vi "Excel___Create Channel Grouping.vi"(0 "Sheets Ref In":refnum<k7>, 5 "Starting Row":i32, 7 "Units String":string, 9 "Action to Perform":u16(ring) items=["", "Start Calibration", "Continue Calibration", "System Initialization", "System Closeout"], 11 "Error In":errorcluster, 12 "Percent Error(F)":bool, 13 "FS(T)/Reading(F)":bool) -> (4 "Sheets Ref Out":refnum<k7>, 15 "Error Out":errorcluster)   [LabVIEW 2019]
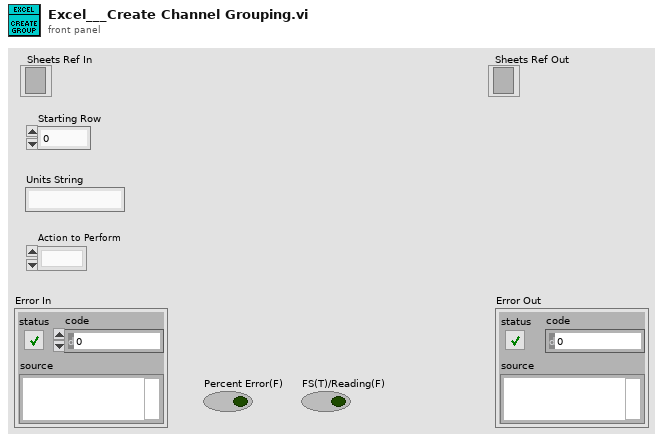
[diagram p1: front panel]
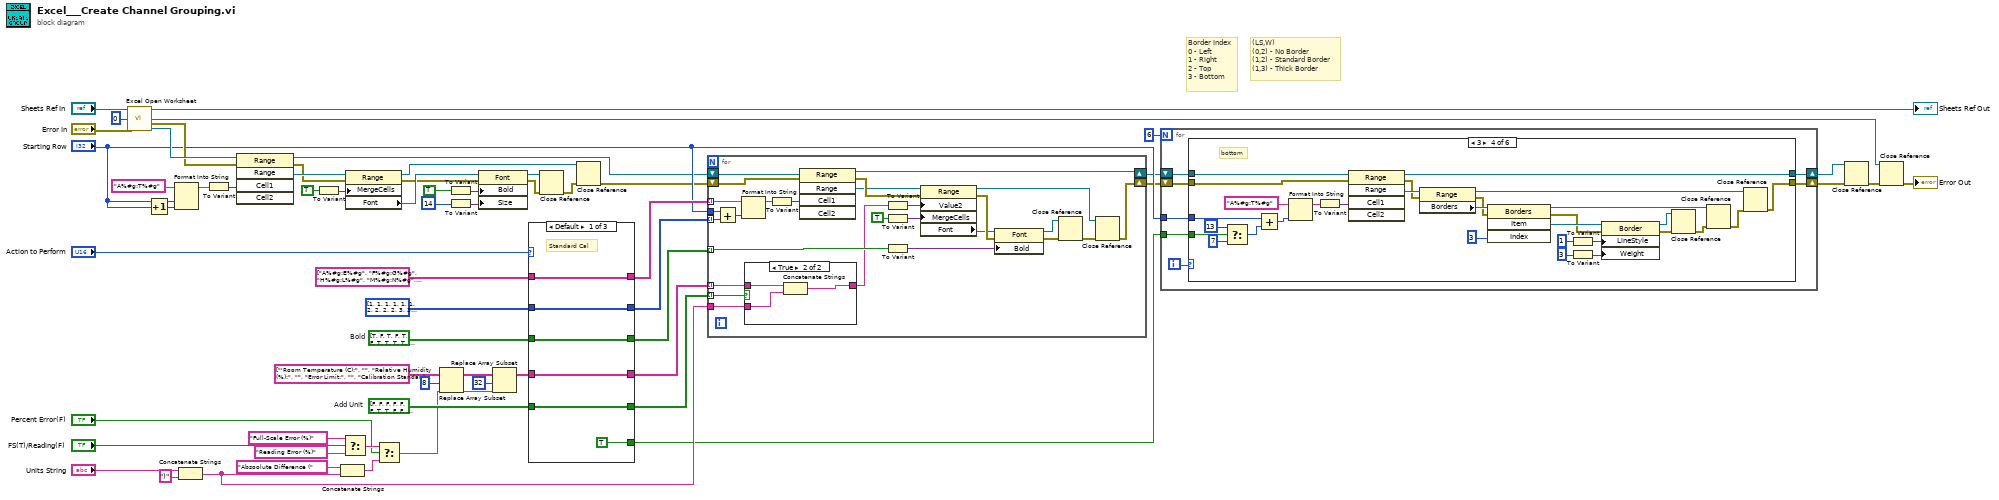
[diagram p0: block diagram]
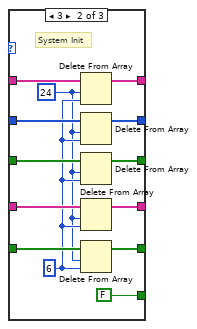
[diagram p3: hidden frame]
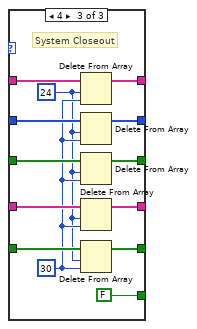
[diagram p4: hidden frame]
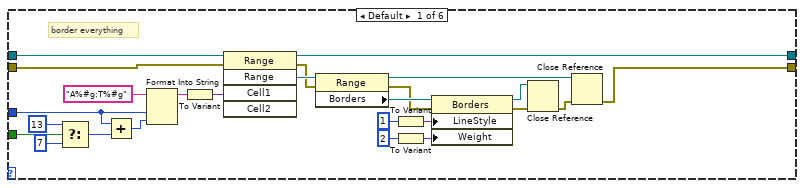
[diagram p5: hidden frame]
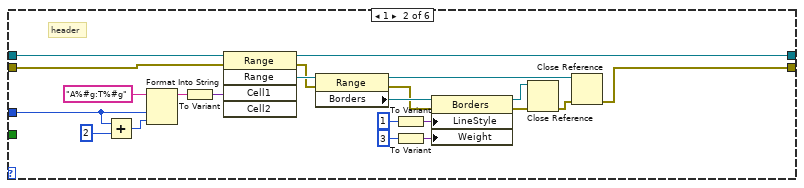
[diagram p6: hidden frame]
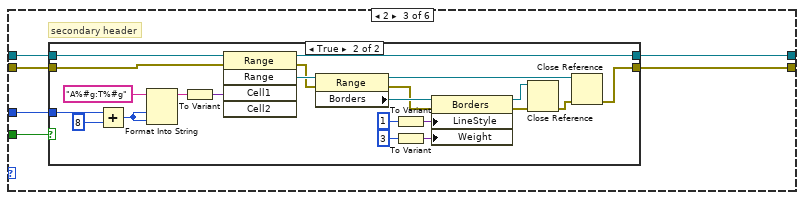
[diagram p7: hidden frame]
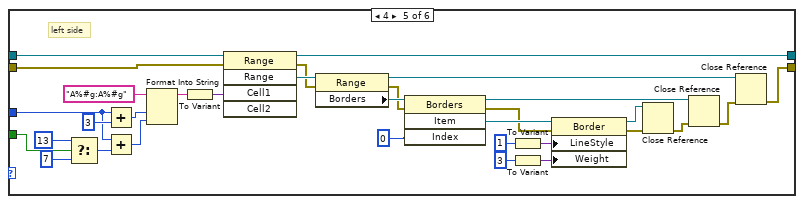
[diagram p9: hidden frame]
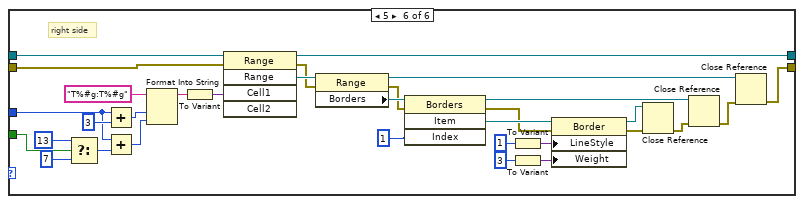
[diagram p10: hidden frame]
diagram:
  w26 = bool[] [FALSE, FALSE, FALSE, FALSE, FALSE, FALSE, TRUE, TRUE, FALSE, FALSE, FALSE, FALSE, FALSE, FALSE, FALSE, FALSE, FALSE, FALSE, FALSE, FALSE, FALSE, FALSE, FALSE, FALSE, FALSE, FALSE, FALSE, FALSE, FALSE, FALSE, TRUE, TRUE, FALSE, FALSE, FALSE, FALSE, FALSE, FALSE, FALSE, FALSE, FALSE, FALSE, FALSE, FALSE, FALSE, FALSE, FALSE, FALSE, FALSE, FALSE, FALSE, FALSE, FALSE, FALSE]  # Add Unit
  w27 = bool[] [TRUE, FALSE, TRUE, FALSE, TRUE, FALSE, TRUE, TRUE, TRUE, TRUE, FALSE, FALSE, FALSE, FALSE, FALSE, FALSE, FALSE, FALSE, FALSE, FALSE, FALSE, FALSE, FALSE, FALSE, FALSE, FALSE, FALSE, FALSE, FALSE, FALSE, TRUE, TRUE, TRUE, TRUE, FALSE, FALSE, FALSE, FALSE, FALSE, FALSE, FALSE, FALSE, FALSE, FALSE, FALSE, FALSE, FALSE, FALSE, FALSE, FALSE, FALSE, FALSE, FALSE, FALSE]  # Bold
  # "(LS,W)\n(0,2) - No Border\n(1,2) - Standard Border\n(1,3) - Thick Border"
  # "Border Index\n0 - Left\n1 - Right\n2 - Top\n3 - Bottom"
  n1 = call "Excel Open Worksheet.vi"("Sheets Ref In"="Sheets Ref In", "Sheet#"=0, "Error In"="Error In") -> ("Sheets Ref Out"=→"Sheets Ref Out":refnum<k7>, "Worksheet Ref Out"=w43:refnum<k7>, "Error Out"=w39:errorcluster, "Cells Ref Out"=w40:refnum<k7>)  [unwired: 9 in]
  n2 = Increment(x="Starting Row") -> (x+1=w61:i32)
  n3 = Format Into String(initial string="A%#g:T%#g", "Starting Row", w61) -> (resulting string=w60:string)  [unwired: 2 in, 1 out]
  n4 = Concatenate Strings("Units String", ")" ("string")) -> (w2:string)
  n5 = To Variant(anything=w60) -> (Variant=w59:variant)
  n6 = invoke class="Range" method="Range"(reference=w40, error in=w39, "Cell1"=w59) -> (reference out=w7:refnum<k7>, error out=w49:errorcluster, "Range"=w58:refnum<k7>)  [unwired: 2 in, 2 out]
  n7 = To Variant(anything=TRUE) -> (Variant=w56:variant)
  n8 = Concatenate Strings("Absoolute Difference (", w2) -> (w15:string)
  n9 = Select(t="Full-Scale Error (%)", s="FS(T)/Reading(F)", f="Reading Error (%)") -> (s? t:f=w16:string)
  n10 = property class="Range"(reference=w58, error in=w49, "MergeCells"=w56) -> (reference out=w34:refnum<k7>, error out=w54:errorcluster, "Font"=w55:refnum<k7>)
  n11 = Select(t=w16, s="Percent Error(F)", f=w15) -> (s? t:f=w14:string)
  n12 = Replace Array Subset(array=string[] ["'Room Temperature (C):", "", "Relative Humidity (%):", "", "Error Limit:", "", "Calibration Standard (", "Reading As Found (", "***placeholder***", "Results", "", "", "", "", "5", "", "", "", "", "10", "", "", "", "", "15", "", "", "", "", "20", "Calibration Standard (", "Reading As Left (", "***placeholder***", "Results", "", "", "", "", "5", "", "", "", "", "10", "", "", "", "", "15", "", "", "", "", "20"], new element=w14, index=8) -> (w13:string[])
  n13 = To Variant(anything=TRUE) -> (Variant=w52:variant)
  n14 = To Variant(anything=14) -> (Variant=w51:variant)
  n15 = property class="Font"(reference=w55, error in=w54, "Bold"=w52, "Size"=w51) -> (reference out=w36:refnum<k7>, error out=w35:errorcluster)
  n16 = Replace Array Subset(array=w13, new element=w14, index=32) -> (w11:string[])
  n17 = case shown="Default" "Action to Perform" {
    tunnel: [w68 w72 w85] -> w25
    tunnel: string[] ["A%#g:E%#g", "F%#g:G%#g", "H%#g:L%#g", "M%#g:N%#g", "O%#g:Q%#g", "R%#g:T%#g", "A%#g:F%#g", "G%#g:L%#g", "M%#g:R%#g", "S%#g:T%#g", "A%#g:F%#g", "G%#g:L%#g", "M%#g:R%#g", "S%#g:T%#g", "A%#g:F%#g", "G%#g:L%#g", "M%#g:R%#g", "S%#g:T%#g", "A%#g:F%#g", "G%#g:L%#g", "M%#g:R%#g", "S%#g:T%#g", "A%#g:F%#g", "G%#g:L%#g", "M%#g:R%#g", "S%#g:T%#g", "A%#g:F%#g", "G%#g:L%#g", "M%#g:R%#g", "S%#g:T%#g", "A%#g:F%#g", "G%#g:L%#g", "M%#g:R%#g", "S%#g:T%#g", "A%#g:F%#g", "G%#g:L%#g", "M%#g:R%#g", "S%#g:T%#g", "A%#g:F%#g", "G%#g:L%#g", "M%#g:R%#g", "S%#g:T%#g", "A%#g:F%#g", "G%#g:L%#g", "M%#g:R%#g", "S%#g:T%#g", "A%#g:F%#g", "G%#g:L%#g", "M%#g:R%#g", "S%#g:T%#g", "A%#g:F%#g", "G%#g:L%#g", "M%#g:R%#g", "S%#g:T%#g"] -> [w68 w76 w94]
    tunnel: [w67 w73 w86] -> w24
    tunnel: i32[] [1, 1, 1, 1, 1, 1, 2, 2, 2, 2, 3, 3, 3, 3, 4, 4, 4, 4, 5, 5, 5, 5, 6, 6, 6, 6, 7, 7, 7, 7, 8, 8, 8, 8, 9, 9, 9, 9, 10, 10, 10, 10, 11, 11, 11, 11, 12, 12, 12, 12, 13, 13, 13, 13] -> [w67 w77 w93]
    tunnel: [w66 w74 w87] -> w22
    tunnel: w27 -> [w66 w78 w92]
    tunnel: [w65 w75 w88] -> w18
    tunnel: w11 -> [w65 w79 w91]
    tunnel: [w64 w80 w89] -> w21
    tunnel: w26 -> [w64 w81 w90]
    tunnel: [TRUE FALSE FALSE] -> w1
    frame Default {
      # "Standard Cal"
    }
    frame 3 {
      w70 = 24 ("length")
      w71 = 6 ("index")
      # "System Init"
      n18 = Delete From Array(array=w76, length=w70, index=w71) -> (array with subset deleted=w72:string[])  [unwired: 1 out]
      n19 = Delete From Array(array=w77, length=w70, index=w71) -> (array with subset deleted=w73:i32[])  [unwired: 1 out]
      n20 = Delete From Array(array=w78, length=w70, index=w71) -> (array with subset deleted=w74:bool[])  [unwired: 1 out]
      n21 = Delete From Array(array=w79, length=w70, index=w71) -> (array with subset deleted=w75:string[])  [unwired: 1 out]
      n22 = Delete From Array(array=w81, length=w70, index=w71) -> (array with subset deleted=w80:bool[])  [unwired: 1 out]
    }
    frame 4 {
      w83 = 24 ("length")
      w84 = 30 ("index")
      # "System Closeout"
      n23 = Delete From Array(array=w94, length=w83, index=w84) -> (array with subset deleted=w85:string[])  [unwired: 1 out]
      n24 = Delete From Array(array=w93, length=w83, index=w84) -> (array with subset deleted=w86:i32[])  [unwired: 1 out]
      n25 = Delete From Array(array=w92, length=w83, index=w84) -> (array with subset deleted=w87:bool[])  [unwired: 1 out]
      n26 = Delete From Array(array=w91, length=w83, index=w84) -> (array with subset deleted=w88:string[])  [unwired: 1 out]
      n27 = Delete From Array(array=w90, length=w83, index=w84) -> (array with subset deleted=w89:bool[])  [unwired: 1 out]
    }
  }
  n28 = Close Reference(reference=w36, error in (no error)=w35) -> (error out=w33:errorcluster)
  n29 = Close Reference(reference=w34, error in (no error)=w33) -> (error out=w6:errorcluster)
  n30 = for {
    tunnel: w25 -> [w121] mode=indexing
    tunnel: "Starting Row" -> [w119]
    tunnel: w24 -> [w118] mode=indexing
    shift-right: [w105] -> w5
    shift-left: w7 -> [w104]
    shift-right: [w103] -> w4
    shift-left: w6 -> [w102]
    tunnel: w22 -> [w99] mode=indexing
    tunnel: w21 -> [w98] mode=indexing
    tunnel: w18 -> [w97] mode=indexing
    tunnel: w2 -> [w95]
    n31 = Add(x=w119, y=w118) -> (x+y=w120:i32)
    n32 = Format Into String(initial string=w121, w120) -> (resulting string=w111:string)  [unwired: 2 in, 1 out]
    n33 = case shown="True" w98 {
      tunnel: w97 -> [w122 w125]
      tunnel: [w122 w124] -> w96
      tunnel: w95 -> [_ w123]
      frame False {
      }
      frame True {
        n34 = Concatenate Strings(w125, w123) -> (w124:string)
      }
    }
    n35 = To Variant(anything=w111) -> (Variant=w112:variant)
    n36 = invoke class="Range" method="Range"(reference=w104, error in=w102, "Cell1"=w112) -> (reference out=w105:refnum<k7>, error out=w117:errorcluster, "Range"=w113:refnum<k7>)  [unwired: 2 in, 2 out]
    n37 = To Variant(anything=w96) -> (Variant=w110:variant)
    n38 = To Variant(anything=TRUE) -> (Variant=w101:variant)
    n39 = To Variant(anything=w99) -> (Variant=w100:variant)
    n40 = property class="Range"(reference=w113, error in=w117, "Value2"=w110, "MergeCells"=w101) -> (reference out=w106:refnum<k7>, error out=w116:errorcluster, "Font"=w115:refnum<k7>)
    n41 = property class="Font"(reference=w115, error in=w116, "Bold"=w100) -> (reference out=w108:refnum<k7>, error out=w109:errorcluster)
    n42 = Close Reference(reference=w108, error in (no error)=w109) -> (error out=w107:errorcluster)
    n43 = Close Reference(reference=w106, error in (no error)=w107) -> (error out=w103:errorcluster)
  }
  n44 = for {
    N: 6 -> [_]
    shift-right: [w132] -> w38
    shift-left: w5 -> [w130]
    tunnel: "Starting Row" -> [w131]
    shift-right: [w129] -> w37
    shift-left: w4 -> [w128]
    tunnel: w1 -> [w126]
    i -> [w127]
    n45 = case shown="3" w127 {
      tunnel: [w155 w178 w185 w239 w269 w301] -> w132
      tunnel: w131 -> [w153 w159 w181 w238 w246 w278]
      tunnel: w130 -> [w151 w177 w184 w237 w267 w299]
      tunnel: [w138 w164 w183 w236 w257 w289] -> w129
      tunnel: w128 -> [w137 w163 w182 w235 w256 w288]
      tunnel: w126 -> [w136 _ w180 w213 w240 w273]
      frame Default {
        # "border everything"
        n46 = Select(t=13 ("y"), s=w136, f=7) -> (s? t:f=w134:i32)
        n47 = Add(x=w153, y=w134) -> (x+y=w154:i32)
        n48 = Format Into String(initial string="A%#g:T%#g", w153, w154) -> (resulting string=w157:string)  [unwired: 2 in, 1 out]
        n49 = To Variant(anything=w157) -> (Variant=w156:variant)
        n50 = invoke class="Range" method="Range"(reference=w151, error in=w137, "Cell1"=w156) -> (reference out=w155:refnum<k7>, error out=w139:errorcluster, "Range"=w150:refnum<k7>)  [unwired: 2 in, 2 out]
        n51 = property class="Range"(reference=w150, error in=w139) -> (reference out=w141:refnum<k7>, error out=w140:errorcluster, "Borders"=w149:refnum<k7>)
        n52 = To Variant(anything=1) -> (Variant=w148:variant)
        n53 = To Variant(anything=2) -> (Variant=w147:variant)
        n54 = property class="Borders"(reference=w149, error in=w140, "LineStyle"=w148, "Weight"=w147) -> (reference out=w142:refnum<k7>, error out=w143:errorcluster)
        n55 = Close Reference(reference=w142, error in (no error)=w143) -> (error out=w144:errorcluster)
        n56 = Close Reference(reference=w141, error in (no error)=w144) -> (error out=w138:errorcluster)
      }
      frame 1 {
        # "header"
        n57 = Add(x=w159, y=2) -> (x+y=w162:i32)
        n58 = Format Into String(initial string="A%#g:T%#g", w159, w162) -> (resulting string=w158:string)  [unwired: 2 in, 1 out]
        n59 = To Variant(anything=w158) -> (Variant=w179:variant)
        n60 = invoke class="Range" method="Range"(reference=w177, error in=w163, "Cell1"=w179) -> (reference out=w178:refnum<k7>, error out=w165:errorcluster, "Range"=w176:refnum<k7>)  [unwired: 2 in, 2 out]
        n61 = property class="Range"(reference=w176, error in=w165) -> (reference out=w167:refnum<k7>, error out=w166:errorcluster, "Borders"=w175:refnum<k7>)
        n62 = To Variant(anything=1) -> (Variant=w174:variant)
        n63 = To Variant(anything=3) -> (Variant=w173:variant)
        n64 = property class="Borders"(reference=w175, error in=w166, "LineStyle"=w174, "Weight"=w173) -> (reference out=w168:refnum<k7>, error out=w169:errorcluster)
        n65 = Close Reference(reference=w168, error in (no error)=w169) -> (error out=w170:errorcluster)
        n66 = Close Reference(reference=w167, error in (no error)=w170) -> (error out=w164:errorcluster)
      }
      frame 2 {
        # "secondary header"
        n67 = case shown="True" w180 {
          tunnel: [w187 w208] -> w185
          tunnel: w184 -> [w187 w207]
          tunnel: [w186 w194] -> w183
          tunnel: w182 -> [w186 w193]
          tunnel: w181 -> [_ w190]
          frame False {
          }
          frame True {
            n68 = Add(x=w190, y=8) -> (x+y=w188:i32)
            n69 = Format Into String(initial string="A%#g:T%#g", w188, w188) -> (resulting string=w189:string)  [unwired: 2 in, 1 out]
            n70 = To Variant(anything=w189) -> (Variant=w209:variant)
            n71 = invoke class="Range" method="Range"(reference=w207, error in=w193, "Cell1"=w209) -> (reference out=w208:refnum<k7>, error out=w195:errorcluster, "Range"=w206:refnum<k7>)  [unwired: 2 in, 2 out]
            n72 = property class="Range"(reference=w206, error in=w195) -> (reference out=w197:refnum<k7>, error out=w196:errorcluster, "Borders"=w205:refnum<k7>)
            n73 = To Variant(anything=1) -> (Variant=w204:variant)
            n74 = To Variant(anything=3) -> (Variant=w203:variant)
            n75 = property class="Borders"(reference=w205, error in=w196, "LineStyle"=w204, "Weight"=w203) -> (reference out=w198:refnum<k7>, error out=w199:errorcluster)
            n76 = Close Reference(reference=w198, error in (no error)=w199) -> (error out=w200:errorcluster)
            n77 = Close Reference(reference=w197, error in (no error)=w200) -> (error out=w194:errorcluster)
          }
        }
      }
      frame 3 {
        # "bottom"
        n78 = Select(t=13 ("y"), s=w213, f=7 ("y")) -> (s? t:f=w210:i32)
        n79 = Add(x=w238, y=w210) -> (x+y=w215:i32)
        n80 = Format Into String(initial string="A%#g:T%#g", w215) -> (resulting string=w234:string)  [unwired: 2 in, 1 out]
        n81 = To Variant(anything=w234) -> (Variant=w233:variant)
        n82 = invoke class="Range" method="Range"(reference=w237, error in=w235, "Cell1"=w233) -> (reference out=w239:refnum<k7>, error out=w223:errorcluster, "Range"=w231:refnum<k7>)  [unwired: 2 in, 2 out]
        n83 = property class="Range"(reference=w231, error in=w223) -> (reference out=w224:refnum<k7>, error out=w220:errorcluster, "Borders"=w222:refnum<k7>)
        n84 = invoke class="Borders" method="Item"(reference=w222, error in=w220, "Index"=3) -> (reference out=w217:refnum<k7>, error out=w214:errorcluster, "Item"=w221:refnum<k7>)  [unwired: 1 in, 1 out]
        n85 = To Variant(anything=1) -> (Variant=w230:variant)
        n86 = To Variant(anything=3) -> (Variant=w229:variant)
        n87 = property class="Border"(reference=w221, error in=w214, "LineStyle"=w230, "Weight"=w229) -> (reference out=w225:refnum<k7>, error out=w226:errorcluster)
        n88 = Close Reference(reference=w225, error in (no error)=w226) -> (error out=w219:errorcluster)
        n89 = Close Reference(reference=w217, error in (no error)=w219) -> (error out=w218:errorcluster)
        n90 = Close Reference(reference=w224, error in (no error)=w218) -> (error out=w236:errorcluster)
      }
      frame 4 {
        # "left side"
        n91 = Select(t=13 ("y"), s=w240, f=7) -> (s? t:f=w242:i32)
        n92 = Add(x=w246, y=3) -> (x+y=w245:i32)
        n93 = Add(x=w246, y=w242) -> (x+y=w248:i32)
        n94 = Format Into String(initial string="A%#g:A%#g", w245, w248) -> (resulting string=w271:string)  [unwired: 2 in, 1 out]
        n95 = To Variant(anything=w271) -> (Variant=w270:variant)
        n96 = invoke class="Range" method="Range"(reference=w267, error in=w256, "Cell1"=w270) -> (reference out=w269:refnum<k7>, error out=w258:errorcluster, "Range"=w266:refnum<k7>)  [unwired: 2 in, 2 out]
        n97 = property class="Range"(reference=w266, error in=w258) -> (reference out=w259:refnum<k7>, error out=w253:errorcluster, "Borders"=w255:refnum<k7>)
        n98 = invoke class="Borders" method="Item"(reference=w255, error in=w253, "Index"=0) -> (reference out=w250:refnum<k7>, error out=w244:errorcluster, "Item"=w254:refnum<k7>)  [unwired: 1 in, 1 out]
        n99 = To Variant(anything=1) -> (Variant=w265:variant)
        n100 = To Variant(anything=3) -> (Variant=w264:variant)
        n101 = property class="Border"(reference=w254, error in=w244, "LineStyle"=w265, "Weight"=w264) -> (reference out=w260:refnum<k7>, error out=w261:errorcluster)
        n102 = Close Reference(reference=w260, error in (no error)=w261) -> (error out=w252:errorcluster)
        n103 = Close Reference(reference=w250, error in (no error)=w252) -> (error out=w251:errorcluster)
        n104 = Close Reference(reference=w259, error in (no error)=w251) -> (error out=w257:errorcluster)
      }
      frame 5 {
        # "right side"
        n105 = Select(t=13 ("y"), s=w273, f=7) -> (s? t:f=w272:i32)
        n106 = Add(x=w278, y=3) -> (x+y=w277:i32)
        n107 = Add(x=w278, y=w272) -> (x+y=w280:i32)
        n108 = Format Into String(initial string="T%#g:T%#g", w277, w280) -> (resulting string=w303:string)  [unwired: 2 in, 1 out]
        n109 = To Variant(anything=w303) -> (Variant=w302:variant)
        n110 = invoke class="Range" method="Range"(reference=w299, error in=w288, "Cell1"=w302) -> (reference out=w301:refnum<k7>, error out=w290:errorcluster, "Range"=w298:refnum<k7>)  [unwired: 2 in, 2 out]
        n111 = property class="Range"(reference=w298, error in=w290) -> (reference out=w291:refnum<k7>, error out=w285:errorcluster, "Borders"=w287:refnum<k7>)
        n112 = invoke class="Borders" method="Item"(reference=w287, error in=w285, "Index"=1) -> (reference out=w282:refnum<k7>, error out=w276:errorcluster, "Item"=w286:refnum<k7>)  [unwired: 1 in, 1 out]
        n113 = To Variant(anything=1) -> (Variant=w297:variant)
        n114 = To Variant(anything=3) -> (Variant=w296:variant)
        n115 = property class="Border"(reference=w286, error in=w276, "LineStyle"=w297, "Weight"=w296) -> (reference out=w292:refnum<k7>, error out=w293:errorcluster)
        n116 = Close Reference(reference=w292, error in (no error)=w293) -> (error out=w284:errorcluster)
        n117 = Close Reference(reference=w282, error in (no error)=w284) -> (error out=w283:errorcluster)
        n118 = Close Reference(reference=w291, error in (no error)=w283) -> (error out=w289:errorcluster)
      }
    }
  }
  n119 = Close Reference(reference=w38, error in (no error)=w37) -> (error out=w44:errorcluster)
  n120 = Close Reference(reference=w43, error in (no error)=w44) -> (error out=→"Error Out":errorcluster)
